vi "jettl Msg Create Queue.vi"(9 "Queue":refnum<class "Queue.lvclass">, 10 "Self Queue Alias":string) -> (2 "Msg Strategy":refnum<class "Msg Strategy.lvclass">)   [LabVIEW 2021, in "Create Queue Msg Strategy.lvlib"]
uses:
  Create Queue Msg Strategy.lvlib
  Create Queue Msg Strategy/Create Queue Msg Strategy.lvclass
  C:/git/jettl/jettl/jettl Msg Create Queue/Create Queue Msg Strategy/Create Queue Msg Strategy.lvclass
  C:/git/jettl/jettl/jettl/Msg Strategy/Msg Strategy.lvclass
  jettl/Queue/Queue.lvclass
  jettl/Msg Strategy/Msg Strategy.lvclass
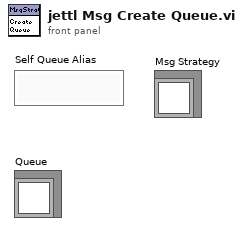
[diagram p1: front panel]
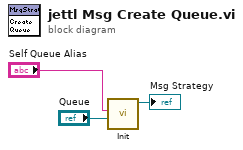
[diagram p0: block diagram]
diagram:
  n1 = call "Init.vi"("Queue"="Queue", "Self Queue Alias"="Self Queue Alias") -> ("Create Queue Msg Strategy out"=→"Msg Strategy":refnum<class "Create Queue Msg Strategy.lvclass">)  [unwired: 9 in]
